vi "06 Temperatura de Equilibrio.vi"() -> ()   [LabVIEW 2021]
panel:
  out "Calor Especifico 2":dbl caption="Calor Específico"
  in  "Material 2":dbl(ring)=0.897 items=["Aluminio"=0.897, "Cobre"=0.385, "Hierro"=0.113, "Plomo"=0.128, "Oro"=0.126, "Mercurio"=0.33, "Plata"=0.233]
  in  "Temperatura 2":dbl caption="Temperatura"
  in  "Masa 2":dbl caption="Masa"
  out "Calor Especifico 1":dbl caption="Calor Específico"
  in  "Material 1":dbl(ring)=0.897 items=["Aluminio"=0.897, "Cobre"=0.385, "Hierro"=0.113, "Plomo"=0.128, "Oro"=0.126, "Mercurio"=0.33, "Plata"=0.233]
  in  "Stop":bool
  out "Temperatura final °C":dbl caption="Temperatura Final:"
  in  "Temperatura 1":dbl caption="Temperatura"
  in  "Masa 1":dbl caption="Masa"
  # "TEMPERATURA DE EQUILIBRIO"
  # "MATERIAL 2"
  # "MATERIAL 1"
  # "g"
  # "g"
  # "°C"
  # "°C"
  # "°C"
  # "Desarrollado por:\n     Semillero Electroquimica e Innovación Ambiental - SEIA"
  # "J"
  # "g °C"
  # "J"
  # "g °C"
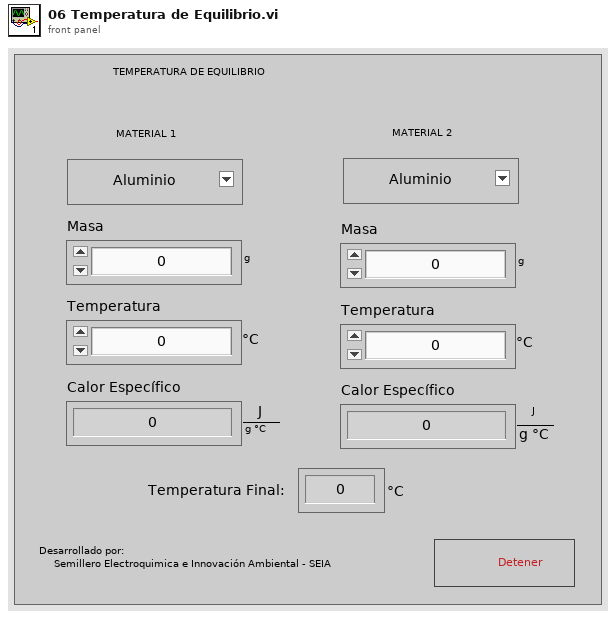
[diagram p1: front panel]
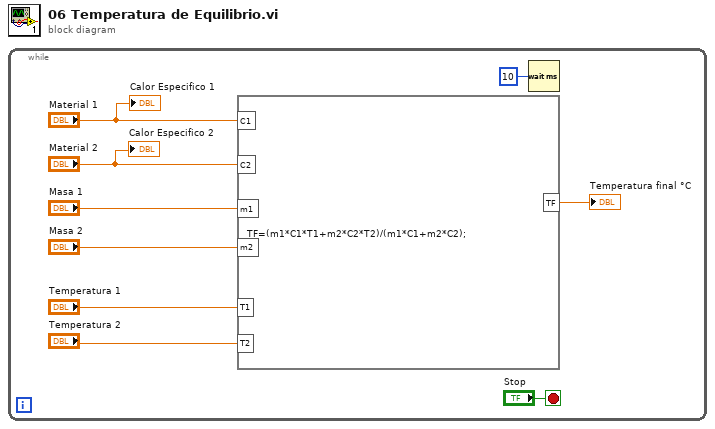
[diagram p0: block diagram]
diagram:
  n1 = while {
    stop <- "Stop" stop-if-true
    n2 = formula code="TF=(m1*C1*T1+m2*C2*T2)/(m1*C1+m2*C2);"("m1"="Masa 1", "C1"="Material 1", "T1"="Temperatura 1", "m2"="Masa 2", "C2"="Material 2", "T2"="Temperatura 2") -> ("TF"=→"Temperatura final °C":dbl)
    n3 = Wait (ms)(milliseconds to wait=u32 10) -> ()  [unwired: 1 out]
    "Calor Especifico 1" <- "Material 1"
    "Calor Especifico 2" <- "Material 2"
  }
